vi "Mouse Down_ on PlotArea.vi"(6 "Coords":T1, 7 "Loop data in":T4={"TitleCollapse"=refnum, "MouseDownState"=enum."Idle", "RightClickCache"={"Mod"={"Ctrl"=FALSE, "Shift"=FALSE}, "CoordsStart"={"Horizontal"=0, "Vertical"=0}, "CoordsEnd"={"Horizontal"=0, "Vertical"=0}, "PlotAreaBounds"={"Left"=10, "Top"=10, "Right"=0, "Bottom"=0}, "slice"=[]}, "ZoomCache"={"SuppressedPlots"=[], "LeftAxis"={"NeedsRevert?"=FALSE, "Scale Fit"=0, "Range"={"Minimum"=0.0, "Maximum"=0.0, "Increment"=0.0, "Minor Increment"=0.0, "Start"=0.0}}, "RightAxis"={"NeedsRevert?"=FALSE, "Scale Fit"=0, "Range"={"Minimum"=0.0, "Maximum"=0.0, "Increment"=0.0, "Minor Increment"=0.0, "Start"=0.0}}, "Mod"={"Shift"=FALSE}}, "UpdateTime"=0.0, "keyboard"=refnum, "visible?"=FALSE}, 8 "error in (no error)":errorcluster, 9 "PlatMods":T3, 10 "ScaleState":T2, 11 "Refs":T13) -> (0 "error out":errorcluster, 5 "Loop data out":T4={"TitleCollapse"=refnum, "MouseDownState"=enum."Idle", "RightClickCache"={"Mod"={"Ctrl"=FALSE, "Shift"=FALSE}, "CoordsStart"={"Horizontal"=0, "Vertical"=0}, "CoordsEnd"={"Horizontal"=0, "Vertical"=0}, "PlotAreaBounds"={"Left"=10, "Top"=10, "Right"=0, "Bottom"=0}, "slice"=[]}, "ZoomCache"={"SuppressedPlots"=[], "LeftAxis"={"NeedsRevert?"=FALSE, "Scale Fit"=0, "Range"={"Minimum"=0.0, "Maximum"=0.0, "Increment"=0.0, "Minor Increment"=0.0, "Start"=0.0}}, "RightAxis"={"NeedsRevert?"=FALSE, "Scale Fit"=0, "Range"={"Minimum"=0.0, "Maximum"=0.0, "Increment"=0.0, "Minor Increment"=0.0, "Start"=0.0}}, "Mod"={"Shift"=FALSE}}, "UpdateTime"=0.0, "keyboard"=refnum, "visible?"=FALSE})   [LabVIEW 2021, in "RocketPlot.lvlib"]
uses:
  RocketPlot.lvlib
  TypeDefs/Plot UI references.ctl
  Classes/RocketPlotHandle/RocketPlotHandle.lvclass
  <userlib>/bjustice/TipStripOOPanel/Classes/TipPanelHandle/TipPanelHandle.lvclass
  TypeDefs/Plot top row.ctl
  TypeDefs/plot while loop data.ctl
  CollapsePanel/CollapsePanel.lvclass
  TypeDefs/MouseDownState.ctl
  TypeDefs/RightClickCache.ctl
  TypeDefs/RightClickCache PlatMod.ctl
  <vilib>/Utility/miscctls.llb/LVPoint32TypeDef.ctl
  <vilib>/Utility/miscctls.llb/LVRectTypeDef.ctl
  TypeDefs/Slice average.ctl
  TypeDefs/ZoomCache.ctl
  TypeDefs/RangeCache.ctl
  <vilib>/Utility/miscctls.llb/LVRangeTypeDef.ctl
  TypeDefs/ZoomCache PlatMod.ctl
  PlatMods to Zoom mods.vi
  Zoom Cache end.vi
  Zoom Cache start.vi
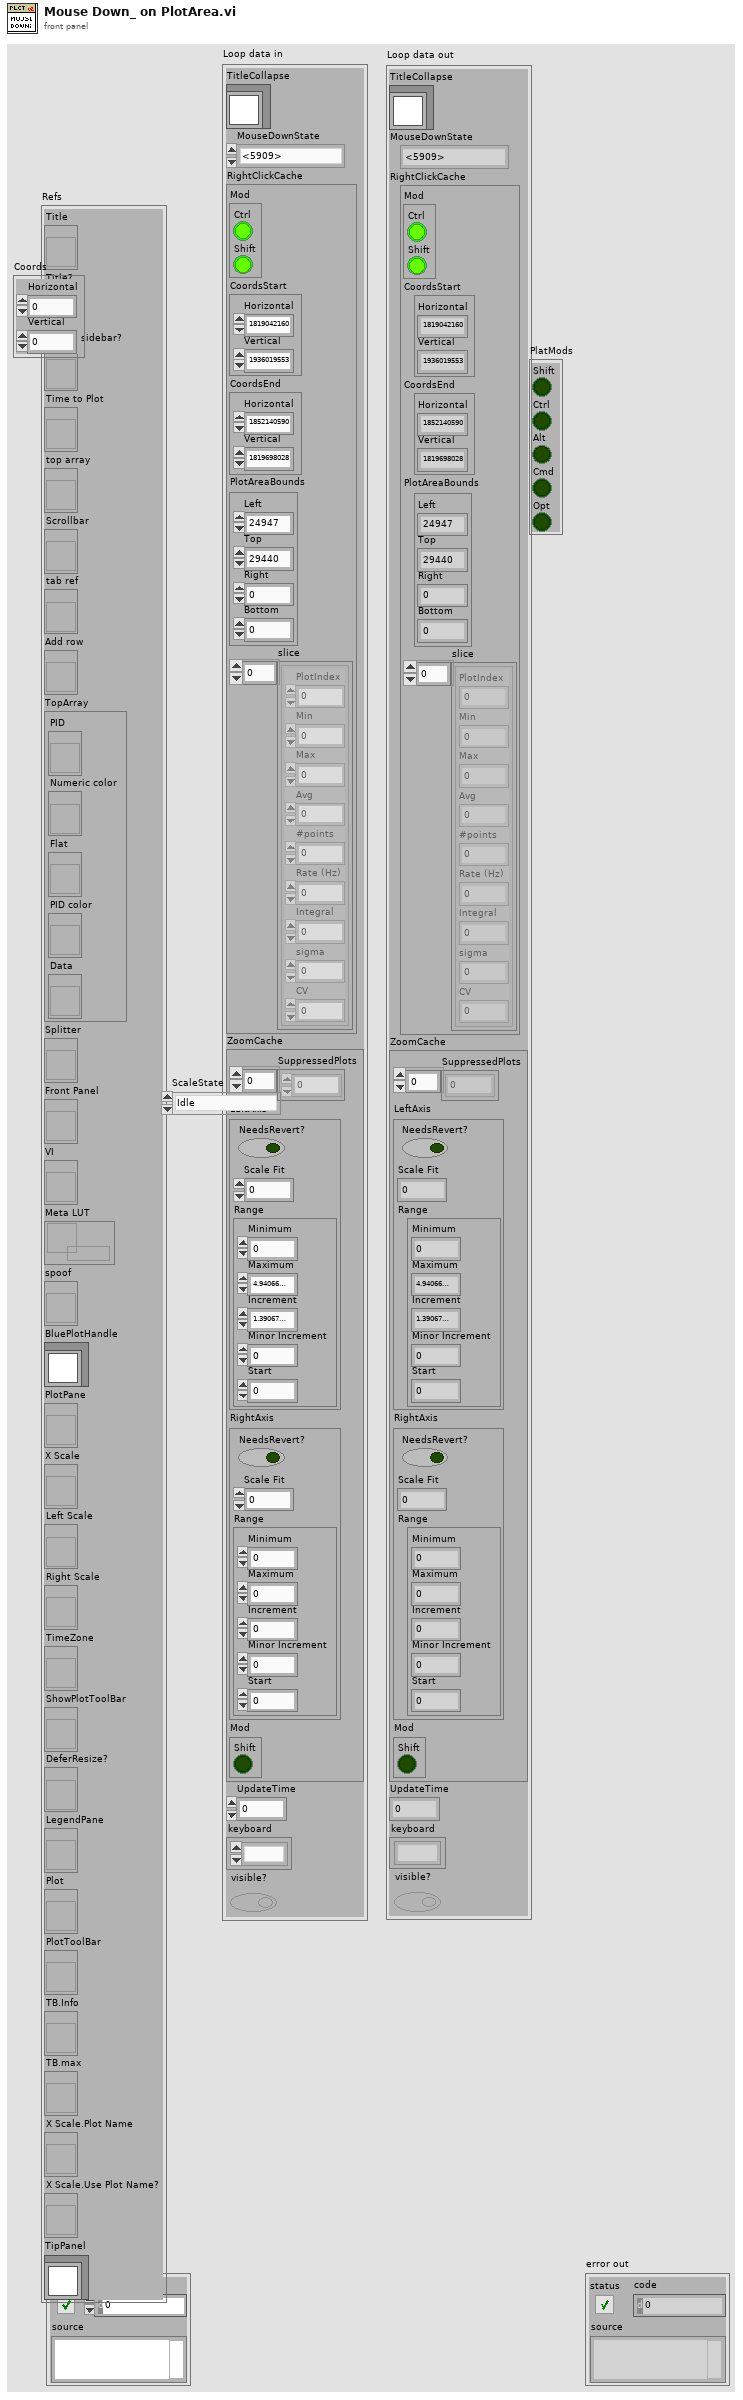
[diagram p1: front panel]
types:
  T1 = typedef "LVPoint32TypeDef.ctl" = cluster{"Horizontal":i32, "Vertical":i32}
  T2 = typedef "RocketPlot.lvlib/MouseDownState.ctl" = enum16{"Idle", "Pan", "Zoom", "Zoom-Post", "RightClick"}
  T3 = cluster{"Shift":bool, "Ctrl":bool, "Alt":bool, "Cmd":bool, "Opt":bool}
  T4 = typedef "RocketPlot.lvlib/plot while loop data.ctl" = cluster{"TitleCollapse":refnum<class "CollapsePanel.lvclass">, "MouseDownState":T2, "RightClickCache":T5, "ZoomCache":T9, "UpdateTime":dbl, "keyboard":refnum<k1>, "visible?":bool}
  T5 = typedef "RocketPlot.lvlib/RightClickCache.ctl" = cluster{"Mod":T6, "CoordsStart":T1, "CoordsEnd":T1, "PlotAreaBounds":T7, "slice":T8[]}
  T6 = typedef "RocketPlot.lvlib/RightClickCache PlatMod.ctl" = cluster{"Ctrl":bool, "Shift":bool}
  T7 = typedef "LVRectTypeDef.ctl" = cluster{"Left":i16, "Top":i16, "Right":i16, "Bottom":i16}
  T8 = typedef "RocketPlot.lvlib/Slice average.ctl" = cluster{"PlotIndex":i32, "Min":dbl, "Max":dbl, "Avg":dbl, "#points":u32, "Rate (Hz)":dbl, "Integral":dbl, "sigma":dbl, "CV":dbl}
  T9 = typedef "RocketPlot.lvlib/ZoomCache.ctl" = cluster{"SuppressedPlots":i32[], "LeftAxis":T10, "RightAxis":T10, "Mod":T12}
  T10 = typedef "RocketPlot.lvlib/RangeCache.ctl" = cluster{"NeedsRevert?":bool, "Scale Fit":u8, "Range":T11}
  T11 = typedef "LVRangeTypeDef.ctl" = cluster{"Minimum":dbl, "Maximum":dbl, "Increment":dbl, "Minor Increment":dbl, "Start":dbl}
  T12 = typedef "RocketPlot.lvlib/ZoomCache PlatMod.ctl" = cluster{"Shift":bool}
  T13 = typedef "RocketPlot.lvlib/Plot UI references.ctl" = cluster{"Title":refnum<vi>, "Title?":refnum<vi>, "Visible sidebar?":refnum<vi>, "Time to Plot":refnum<vi>, "top array":refnum<vi>, "Scrollbar":refnum<vi>, "tab ref":refnum<vi>, "Add row":refnum<vi>, "TopArray":cluster{"PID":refnum<vi>, "Numeric color":refnum<vi>, "Flat":refnum<vi>, "PID color":refnum<vi>, "Data":refnum<vi>}, "Splitter":refnum<vi>, "Front Panel":refnum<vi>, "VI":refnum<vi>, "Meta LUT":refnum<data-value>, "spoof":refnum<vi>, "BluePlotHandle":refnum<class "RocketPlotHandle.lvclass">, "PlotPane":refnum<vi>, "X Scale":refnum<vi>, "Left Scale":refnum<vi>, "Right Scale":refnum<vi>, "TimeZone":refnum<vi>, "ShowPlotToolBar":refnum<vi>, "DeferResize?":refnum<vi>, "LegendPane":refnum<vi>, "Plot":refnum<vi>, "PlotToolBar":refnum<vi>, "TB.Info":refnum<vi>, "TB.max":refnum<vi>, "X Scale.Plot Name":refnum<vi>, "X Scale.Use Plot Name?":refnum<vi>, "TipPanel":refnum<class "TipPanelHandle.lvclass">}
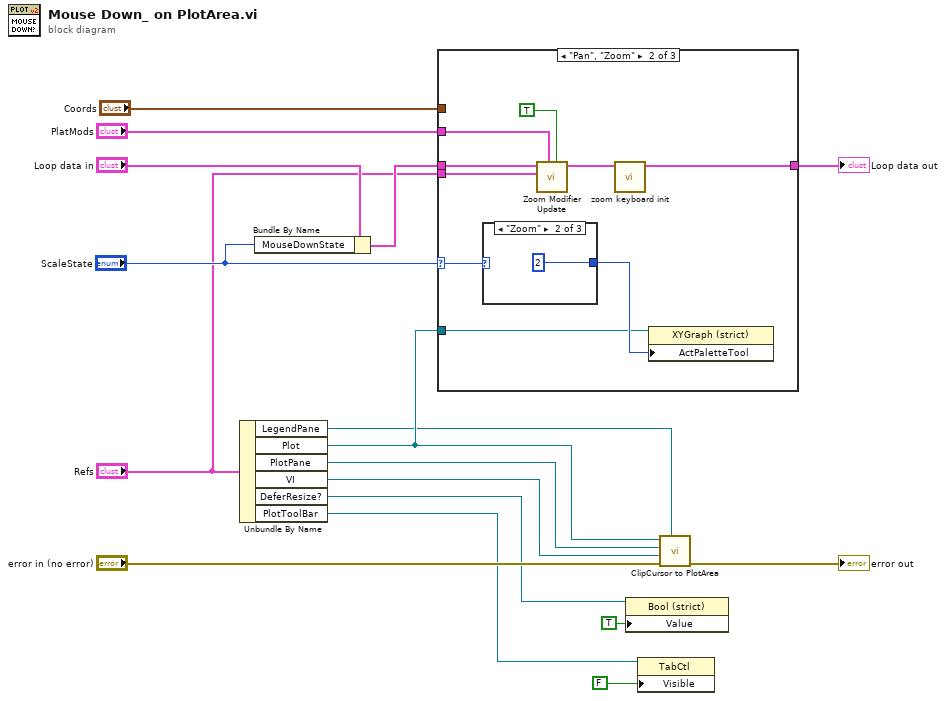
[diagram p0: block diagram]
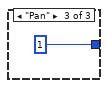
[diagram p4: hidden frame]
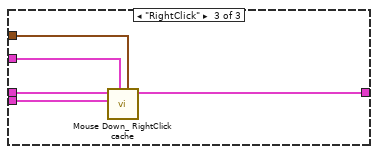
[diagram p5: hidden frame]
diagram:
  n1 = Unbundle By Name("Refs") -> ("LegendPane"=w8:refnum<vi>, "Plot"=w9:refnum<vi>, "PlotPane"=w14:refnum<vi>, "VI"=w13:refnum<vi>, "DeferResize?"=w11:refnum<vi>, "PlotToolBar"=w2:refnum<vi>)
  n2 = Bundle By Name(cluster="Loop data in", "MouseDownState"="ScaleState") -> (w5:T4)
  n3 = case shown="\"Pan\", \"Zoom\"" "ScaleState" {
    selector: "ScaleState" -> [_ w25 _]
    tunnel: w5 -> [w18 w24 w34]
    tunnel: [w18 w19 w33] -> w12
    tunnel: "Refs" -> [_ w22 w32]
    tunnel: "PlatMods" -> [_ w23 w31]
    tunnel: w9 -> [_ w26 _]
    tunnel: "Coords" -> [_ _ w30]
    frame Default {
    }
    frame "Pan", "Zoom" {
      n4 = case shown="\"Zoom\"" w25 {
        tunnel: [_ 2 ("Palette:Active Tool") 1 ("Palette:Active Tool")] -> w27
        frame Default {
        }
        frame "Zoom" {
        }
        frame "Pan" {
        }
      }
      n5 = call "Zoom Modifier Update.vi"("Start new?"=TRUE ("Force update?"), "PlatMods"=w23, "Refs"=w22, "Loop data in"=w24) -> ("Loop data out"=w20:T4)  [unwired: 6 in, 1 out]
      n6 = call "zoom keyboard init.vi"("Loop data in"=w20) -> ("Loop data out"=w19:T4)  [unwired: 9 in, 1 out]
      n7 = property class="XYGraph (strict)"(reference=w26, "ActPaletteTool"=w27) -> ()  [unwired: 1 in, 2 out]
    }
    frame "RightClick" {
      n8 = call "Mouse Down_ RightClick cache.vi"("Coords"=w30, "PlatMods"=w31, "Refs"=w32, "Loop data in"=w34) -> ("Loop data out"=w33:T4)  [unwired: 6 in, 1 out]
    }
  }
  "Loop data out" <- w12
  n9 = property class="Bool (strict)"(reference=w11, "Value"=TRUE) -> ()  [unwired: 1 in, 2 out]
  n10 = property class="TabCtl"(reference=w2, "Visible"=FALSE) -> ()  [unwired: 1 in, 2 out]
  n11 = call "ClipCursor to PlotArea.vi"("OriginPane"=w8, "error in (no error)"="error in (no error)", "VI"=w13, "PlotPane"=w14, "plot ref"=w9) -> ("error out"=→"error out":errorcluster)  [unwired: 6 in]
